vi "TimeOut_03.vi"(3 "error in (no error)":errorcluster, 4 "Reset":bool) -> (0 "error out":errorcluster)   [LabVIEW 2011]
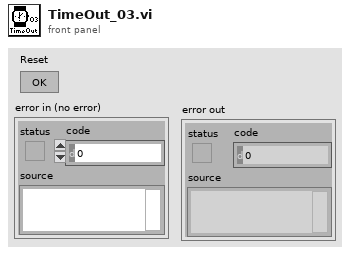
[diagram p1: front panel]
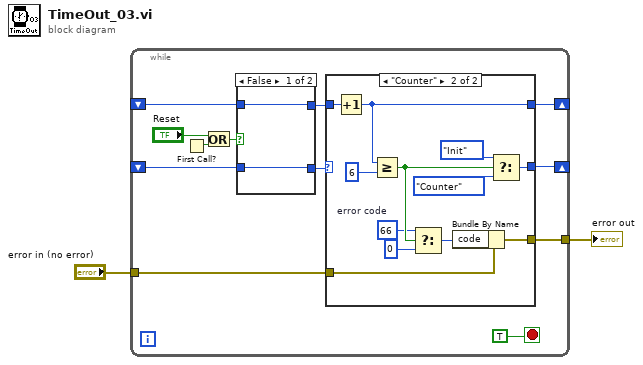
[diagram p0: block diagram]
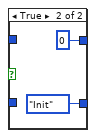
[diagram p2: hidden frame]
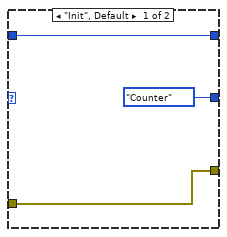
[diagram p3: hidden frame]
diagram:
  n1 = while {
    shift-right: [w14] -> _
    shift-left: _ -> [w9]
    shift-right: [w13] -> _
    shift-left: _ -> [w8]
    tunnel: "error in (no error)" -> [w4]
    tunnel: [w3] -> w1
    stop <- TRUE stop-if-true
    n2 = First Call?() -> (First Call?: T/F=w5:bool)
    n3 = Or(x="Reset", y=w5) -> (x .or. y?=w7:bool)
    n4 = case shown="False" w7 {
      tunnel: [w15 enum16{"Init", "Counter"}."Init" ("Enum")] -> w10
      tunnel: [w16 u8 0 ("y")] -> w11
      tunnel: w9 -> [w16 _]
      tunnel: w8 -> [w15 _]
      frame False {
      }
      frame True {
      }
    }
    n5 = case shown="\"Counter\"" w10 {
      tunnel: [w20 w32] -> w14
      tunnel: w11 -> [w20 w33]
      tunnel: [enum16{"Init", "Counter"}."Counter" ("Enum") w29] -> w13
      tunnel: w4 -> [w19 w22]
      tunnel: [w19 w28] -> w3
      frame "Init", Default {
      }
      frame "Counter" {
        w25 = 66  # error code
        n6 = Increment(x=w33) -> (x+1=w32:u8)
        n7 = Greater Or Equal?(x=w32, y=u8 6) -> (x >= y?=w26:bool)
        n8 = Select(t=w25, s=w26, f=0) -> (s? t:f=w23:i32)
        n9 = Bundle By Name(cluster=w22, "code"=w23) -> (w28:errorcluster)
        n10 = Select(t=enum16{"Init", "Counter"}."Init" ("Enum"), s=w26, f=enum16{"Init", "Counter"}."Counter" ("Enum")) -> (s? t:f=w29:enum16{"Init", "Counter"})
      }
    }
  }
  "error out" <- w1
